vi "Ends With.vi"(10 "String":string, 11 "Suffix":string) -> (2 "String length":i32, 3 "Ended with":bool)   [LabVIEW 2020, in "LV Tiff.lvlib"]
uses:
  LV Tiff.lvlib
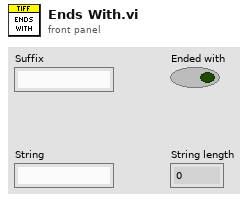
[diagram p1: front panel]
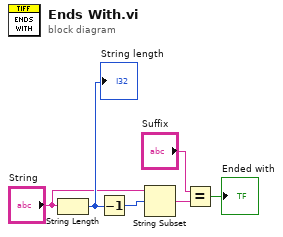
[diagram p0: block diagram]
diagram:
  n1 = String Length(string="String") -> (length=w6:i32)
  "String length" <- w6
  n2 = Decrement(x=w6) -> (x-1=w2:i32)
  n3 = String Subset(string="String", offset (0)=w2) -> (substring=w3:string)  [unwired: 1 in]
  n4 = Equal?(x="Suffix", y=w3) -> (x = y?=→"Ended with":bool)
